vi "Cal_Timeout.vi"   [LabVIEW 2017]
uses:
  Custom Controls/scan mode main settings tab.ctl
  GFG/GFGnumericGet.vi
  GFG/GFGfpRefGet.vi
  GFG/GFGbooleanGet.vi
  GFG/GFG library.lvlib
types:
  T1 = typedef "scan mode main settings tab.ctl" = enum32{"2D frame", "2D line scan", "general settings", "Z Stack", "piezo"}
  T2 = cluster{"WaveformChartRef":refnum<vi>, "DigitalRef":refnum<vi>, "ArrayRef":refnum<vi>, "TabControlRef":refnum<vi>, "EnumRef":refnum<vi>, "RingRef":refnum<vi>, "BooleanRef":refnum<vi>, "KnobRef":refnum<vi>, "SlideRef":refnum<vi>, "PathRef":refnum<vi>, "StringRef":refnum<vi>, "ComboBox":refnum<vi>, "WaveformGraphRef":refnum<vi>}
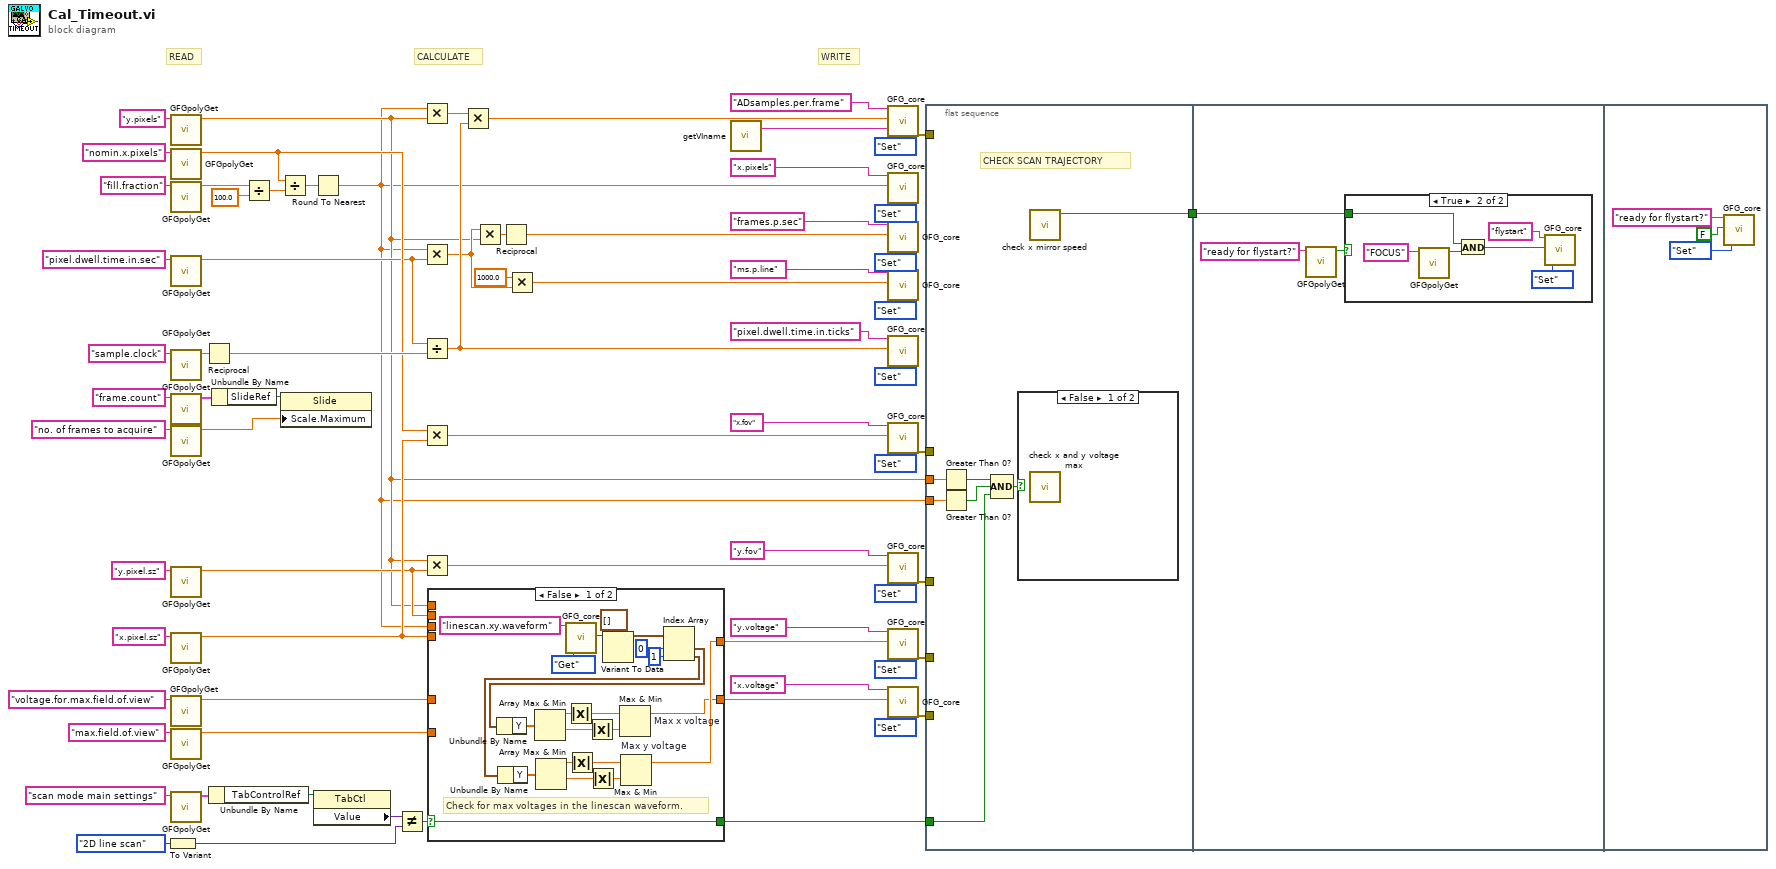
[diagram p0: block diagram]
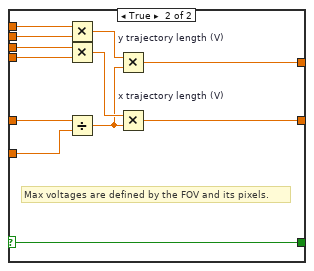
[diagram p2: hidden frame]
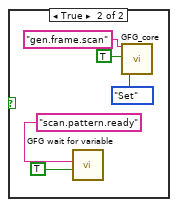
[diagram p3: hidden frame]
diagram:
  # "WRITE"
  # "CALCULATE"
  # "READ"
  n1 = To Variant(anything=scan_mode_main_settings_tab."2D line scan" ("scan mode main settings")) -> (Variant=w4:variant)
  n2 = call-poly "GFGpolyGet.vi"("Variable Name in"="y.pixels") -> ("Numeric"=w11:dbl)  [unwired: 8 in, 2 out]
  n3 = call-poly "GFGpolyGet.vi"("Variable Name in"="nomin.x.pixels") -> ("Numeric"=w33:dbl)  [unwired: 8 in, 2 out]
  n4 = call-poly "GFGpolyGet.vi"("Variable Name in"="fill.fraction") -> ("Numeric"=w53:dbl)  [unwired: 8 in, 2 out]
  n5 = call-poly "GFGpolyGet.vi"("Variable Name in"="pixel.dwell.time.in.sec") -> ("Numeric"=w25:dbl)  [unwired: 8 in, 2 out]
  n6 = call-poly "GFGpolyGet.vi"("Variable Name in"="sample.clock") -> ("Numeric"=w35:dbl)  [unwired: 8 in, 2 out]
  n7 = call-poly "GFGpolyGet.vi"("Variable Name in"="frame.count") -> ("output cluster"=w20:T2)  [unwired: 9 in, 1 out]
  n8 = call-poly "GFGpolyGet.vi"("Variable Name in"="no. of frames to acquire") -> ("Numeric"=w17:dbl)  [unwired: 8 in, 2 out]
  n9 = call-poly "GFGpolyGet.vi"("Variable Name in"="y.pixel.sz") -> ("Numeric"=w36:dbl)  [unwired: 8 in, 2 out]
  n10 = call-poly "GFGpolyGet.vi"("Variable Name in"="x.pixel.sz") -> ("Numeric"=w37:dbl)  [unwired: 8 in, 2 out]
  n11 = call-poly "GFGpolyGet.vi"("Variable Name in"="voltage.for.max.field.of.view") -> ("Numeric"=w44:dbl)  [unwired: 8 in, 2 out]
  n12 = call-poly "GFGpolyGet.vi"("Variable Name in"="max.field.of.view") -> ("Numeric"=w45:dbl)  [unwired: 8 in, 2 out]
  n13 = call-poly "GFGpolyGet.vi"("Variable Name in"="scan mode main settings") -> ("output cluster"=w8:T2)  [unwired: 9 in, 1 out]
  n14 = Reciprocal(x=w35) -> (1/x=w60:dbl)
  n15 = Unbundle By Name(w8) -> ("TabControlRef"=w6:refnum<vi>)
  n16 = Unbundle By Name(w20) -> ("SlideRef"=w19:refnum<vi>)
  n17 = Divide(x=w53, y=100.0) -> (x/y=w49:dbl)
  n18 = Divide(x=w33, y=w49) -> (x/y=w34:dbl)
  n19 = property class="Slide"(reference=w19, "Scale.Maximum"=w17) -> ()  [unwired: 1 in, 2 out]
  n20 = Round To Nearest(number=w34) -> (nearest integer value=w10:dbl)
  n21 = property class="TabCtl"(reference=w6) -> ("Value"=w3:variant)  [unwired: 1 in, 2 out]
  n22 = Not Equal?(x=w3, y=w4) -> (x != y?=w2:bool)
  n23 = Multiply(x=w10, y=w11) -> (x*y=w32:dbl)
  n24 = Multiply(x=w10, y=w25) -> (x*y=w24:dbl)
  n25 = Divide(x=w25, y=w60) -> (x/y=w56:dbl)
  n26 = Multiply(x=w33, y=w37) -> (x*y=w65:dbl)
  n27 = Multiply(x=w11, y=w36) -> (x*y=w62:dbl)
  n28 = case shown="False" w2 {
    selector: w2 -> [w95 w96]
    tunnel: w45 -> [_ w107]
    tunnel: w44 -> [_ w106]
    tunnel: [w74 w105] -> w39
    tunnel: [w75 w104] -> w38
    tunnel: w37 -> [_ w103]
    tunnel: w36 -> [_ w101]
    tunnel: w11 -> [_ w100]
    tunnel: w10 -> [_ w99]
    tunnel: [w95 w96] -> w1
    frame False {
      # "Check for max voltages in the linescan waveform."
      n29 = call "GFG_core.vi"("Variable Name in"="linescan.xy.waveform", "Action"=enum16{"Init", "Set", "Get"}."Get") -> ("Variant Out"=w79:variant)  [unwired: 11 in, 6 out]
      n30 = Variant To Data(type=waveform(dbl)[] [] ("appended array"), Variant=w79) -> (data=w80:waveform(dbl)[])  [unwired: 1 in, 1 out]
      n31 = Index Array(array=w80, index #1=0 ("index"), index #2=1 ("index")) -> (element #1=w83:waveform(dbl), element #2=w84:waveform(dbl))
      n32 = Unbundle By Name(w83) -> ("Y"=w85:dbl[])
      n33 = Unbundle By Name(w84) -> ("Y"=w94:dbl[])
      n34 = Array Max & Min(array=w85) -> (max value=w86:dbl, min value=w87:dbl)  [unwired: 2 out]
      n35 = Array Max & Min(array=w94) -> (max value=w93:dbl, min value=w92:dbl)  [unwired: 2 out]
      n36 = Absolute Value(x=w86) -> (abs(x)=w88:dbl)
      n37 = Absolute Value(x=w93) -> (abs(x)=w91:dbl)
      n38 = Absolute Value(x=w87) -> (abs(x)=w89:dbl)
      n39 = Absolute Value(x=w92) -> (abs(x)=w90:dbl)
      n40 = Max & Min "Max x voltage"(x=w88, y=w89) -> (max(x,y)=w74:dbl)  [unwired: 1 out]
      n41 = Max & Min "Max y voltage"(x=w91, y=w90) -> (max(x,y)=w75:dbl)  [unwired: 1 out]
    }
    frame True {
      # "Max voltages are defined by the FOV and its pixels."
      n42 = Multiply(x=w100, y=w101) -> (x*y=w97:dbl)
      n43 = Multiply(x=w99, y=w103) -> (x*y=w102:dbl)
      n44 = Divide(x=w106, y=w107) -> (x/y=w98:dbl)
      n45 = Multiply "y trajectory length (V)"(x=w97, y=w98) -> (x*y=w104:dbl)
      n46 = Multiply "x trajectory length (V)"(x=w102, y=w98) -> (x*y=w105:dbl)
    }
  }
  n47 = Multiply(x=w32, y=w56) -> (x*y=w71:dbl)
  n48 = Multiply(x=w24, y=w11) -> (x*y=w27:dbl)
  n49 = Reciprocal(x=w27) -> (1/x=w26:dbl)
  n50 = Multiply(x=1000.0, y=w24) -> (x*y=w22:dbl)
  n51 = call "getVIname.vi"() -> ("VI name"=w69:string)  [unwired: 19 in]
  n52 = call "GFG_core.vi"("Variable Name in"="ADsamples.per.frame", "Variant in"=w71, "Source VI"=w69, "Action"=enum16{"Init", "Set", "Get"}."Set") -> ("error out"=w16:errorcluster)  [unwired: 9 in, 6 out]
  n53 = call "GFG_core.vi"("Variable Name in"="x.pixels", "Variant in"=w10, "Action"=enum16{"Init", "Set", "Get"}."Set") -> ()  [unwired: 10 in, 7 out]
  n54 = call "GFG_core.vi"("Variable Name in"="frames.p.sec", "Variant in"=w26, "Action"=enum16{"Init", "Set", "Get"}."Set") -> ()  [unwired: 10 in, 7 out]
  n55 = call "GFG_core.vi"("Variable Name in"="ms.p.line", "Variant in"=w22, "Action"=enum16{"Init", "Set", "Get"}."Set") -> ()  [unwired: 10 in, 7 out]
  n56 = call "GFG_core.vi"("Variable Name in"="pixel.dwell.time.in.ticks", "Variant in"=w56, "Action"=enum16{"Init", "Set", "Get"}."Set") -> ()  [unwired: 10 in, 7 out]
  n57 = call "GFG_core.vi"("Variable Name in"="x.fov", "Variant in"=w65, "Action"=enum16{"Init", "Set", "Get"}."Set") -> ("error out"=w15:errorcluster)  [unwired: 10 in, 6 out]
  n58 = call "GFG_core.vi"("Variable Name in"="y.fov", "Variant in"=w62, "Action"=enum16{"Init", "Set", "Get"}."Set") -> ("error out"=w14:errorcluster)  [unwired: 10 in, 6 out]
  n59 = call "GFG_core.vi"("Variable Name in"="y.voltage", "Variant in"=w38, "Action"=enum16{"Init", "Set", "Get"}."Set") -> ("error out"=w13:errorcluster)  [unwired: 10 in, 6 out]
  n60 = call "GFG_core.vi"("Variable Name in"="x.voltage", "Variant in"=w39, "Action"=enum16{"Init", "Set", "Get"}."Set") -> ("error out"=w12:errorcluster)  [unwired: 10 in, 6 out]
  n61 = flat-sequence {
    tunnel: w16 -> [_]
    tunnel: w15 -> [_]
    tunnel: w14 -> [_]
    tunnel: w13 -> [_]
    tunnel: w12 -> [_]
    tunnel: [w114] -> w73
    tunnel: w11 -> [w112]
    tunnel: w10 -> [w109]
    tunnel: w1 -> [w108]
    tunnel: w73 -> [w122]
    frame #0 {
      # "CHECK SCAN TRAJECTORY"
      n62 = Greater Than 0?(x=w112) -> (x > 0?=w111:bool)
      n63 = Greater Than 0?(x=w109) -> (x > 0?=w110:bool)
      n64 = Compound Arithmetic op=AND(w111, w110, w108) -> (w113:bool)
      n65 = case shown="False" w113 {
        frame False {
          n66 = call "check x and y voltage max.vi"() -> ()  [unwired: 11 in, 1 out]
        }
        frame True {
          n67 = call "GFG wait for variable.vi"("Variant"=TRUE, "Variable Name"="scan.pattern.ready" ("Variable Name in")) -> ()  [unwired: 10 in]
          n68 = call "GFG_core.vi"("Variable Name in"="gen.frame.scan", "Variant in"=TRUE, "Action"=enum16{"Init", "Set", "Get"}."Set") -> ()  [unwired: 10 in, 7 out]
        }
      }
      n69 = call "check x mirror speed.vi"() -> ("mirror speed valid"=w114:bool)  [unwired: 11 in]
    }
    frame #1 {
      n70 = call-poly "GFGpolyGet.vi"("Variable Name in"="ready for flystart?") -> ("Boolean Value OUT"=w120:bool)  [unwired: 9 in, 1 out]
      n71 = case shown="True" w120 {
        tunnel: w122 -> [_ w125]
        frame False {
        }
        frame True {
          n72 = call-poly "GFGpolyGet.vi"("Variable Name in"="FOCUS") -> ("Boolean Value OUT"=w127:bool)  [unwired: 9 in, 1 out]
          n73 = And(x=w125, y=w127) -> (x .and. y?=w126:bool)
          n74 = call "GFG_core.vi"("Variable Name in"="flystart", "Variant in"=w126, "Action"=enum16{"Init", "Set", "Get"}."Set") -> ()  [unwired: 10 in, 7 out]
        }
      }
    }
    frame #2 {
      n75 = call "GFG_core.vi"("Variable Name in"="ready for flystart?", "Variant in"=FALSE ("ready for flystart?"), "Action"=enum16{"Init", "Set", "Get"}."Set") -> ()  [unwired: 10 in, 7 out]
    }
  }
